vi "Teleop.vi"(10 "Match Info":T1={"Autonomous Elapsed Seconds"=0.0, "TeleOp Elapsed Seconds"=27.581, "Disabled Elapsed Seconds"=153.74, "Visited Autonomous"=FALSE, "Visited TeleOp"=TRUE, "Visited Disabled"=TRUE, "Autonomous Settings"={"Autonomous Style"=enum."Independent", "VI Refnum"=refnum}}, 11 "Call Context":T2=enum."Stop") -> ()   [LabVIEW 2017]
doc: "This VI is called for each enabled TeleOp packet received from the DS. It is typically used to read from joysticks and other inputs and update I/O or setpoints for timed control loops. It should complete and return within 20 milliseconds or risk missing DS packets."
uses:
  <vilib>/Rock Robotics/WPI/DriverStation/WPI_DriverStationDerivedRobotMode.ctl
  <vilib>/Rock Robotics/WPI/DriverStation/WPI_DriverStationMatch Info.ctl
  <vilib>/Rock Robotics/WPI/Utilities/WPI_GetSetVariantRefNum.vi
  Elevator/Implementation/Elevator Published Globals.vi
  <vilib>/Rock Robotics/Network Tables/NT Write Boolean.vi
  Framework/Robot Global Data.vi
  Configuration/Constants.vi
  <vilib>/Rock Robotics/Network Tables/NT Write Numeric Array.vi
  <vilib>/Rock Robotics/Network Tables/NT Write Boolean Array.vi
panel:
  in  "ElevatorheightToSLowMode":dbl=25.0 format="%#_13g"
  in  "OutakeSpeed Fast":dbl=-1.0 format="%#_13g"
  in  "ElevatorInterpolate":cluster{"X":dbl, "Y":dbl}[](array[cluster])=[{"X"=0.0, "Y"=0.0}, {"X"=0.05, "Y"=0.0}, {"X"=0.8, "Y"=0.3}, {"X"=1.0, "Y"=1.0}]
  in  "DisableElevatorSpeed":dbl
  in  "OutakeSens":dbl=0.7
  in  "ElevatorheightToSLowerMode":dbl=45.0 format="%#_13g"
  in  "OutakeSpeed":dbl=-0.7 format="%#_13g"
  in  "IntakeDeadbandFOrOutakeingForTime":dbl=0.06
  in  "Intake Sens":dbl=1.2
  in  "Max dx/dt":dbl=100.0
  in  "Points":cluster{"X":dbl, "Y":dbl}[](array[cluster])=[{"X"=0.0, "Y"=0.0}, {"X"=0.02, "Y"=0.0}, {"X"=0.021, "Y"=0.15}, {"X"=1.0, "Y"=1.0}]
  in  "Drive":enum16{"Cheesy", "Tank"}(ring)
  # "Keep negative"
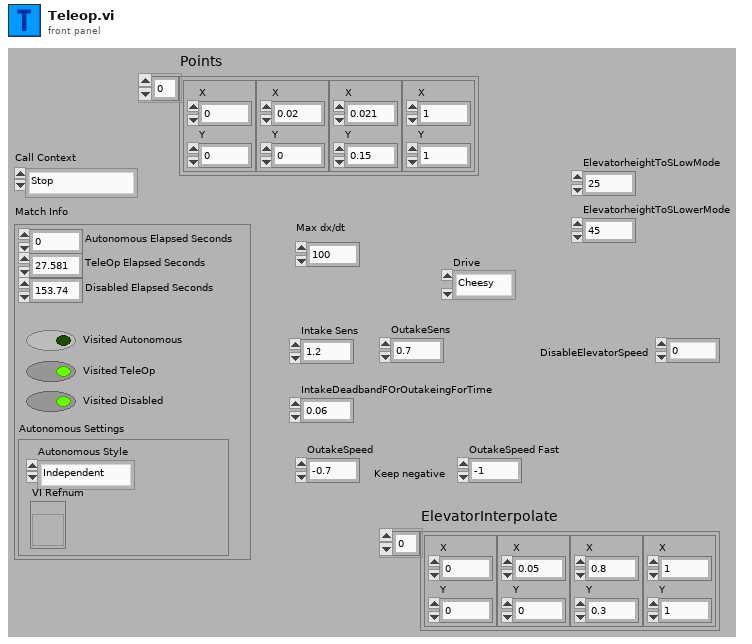
[diagram p1: front panel]
types:
  T1 = typedef "WPI_DriverStationMatch Info.ctl" = cluster{"Autonomous Elapsed Seconds":dbl, "TeleOp Elapsed Seconds":dbl, "Disabled Elapsed Seconds":dbl, "Visited Autonomous":bool, "Visited TeleOp":bool, "Visited Disabled":bool, "Autonomous Settings":cluster{"Autonomous Style":enum16{"Iterative", "Independent"}, "VI Refnum":refnum<vi>}}
  T2 = typedef "WPI_DriverStationDerivedRobotMode.ctl" = enum16{"Init", "Execute", "Stop"}
  T3 = typedef "WPI_JoystickDevRef.ctl" = cluster{"Device":T4}
  T4 = typedef "WPI_JoystickDeviceEnum.ctl" = enum16{"USB 0", "USB 1", "USB 2", "USB 3", "USB 4", "USB 5"}
  T5 = typedef "Command Status Info.ctl" = cluster{"Name":string, "Status":T6, "notifier out":T7}
  T6 = typedef "Completion Status.ctl" = enum16{"Successful", "Aborted", "Incomplete"}
  T7 = typedef "Completion Notifier.ctl" = refnum<notifier>
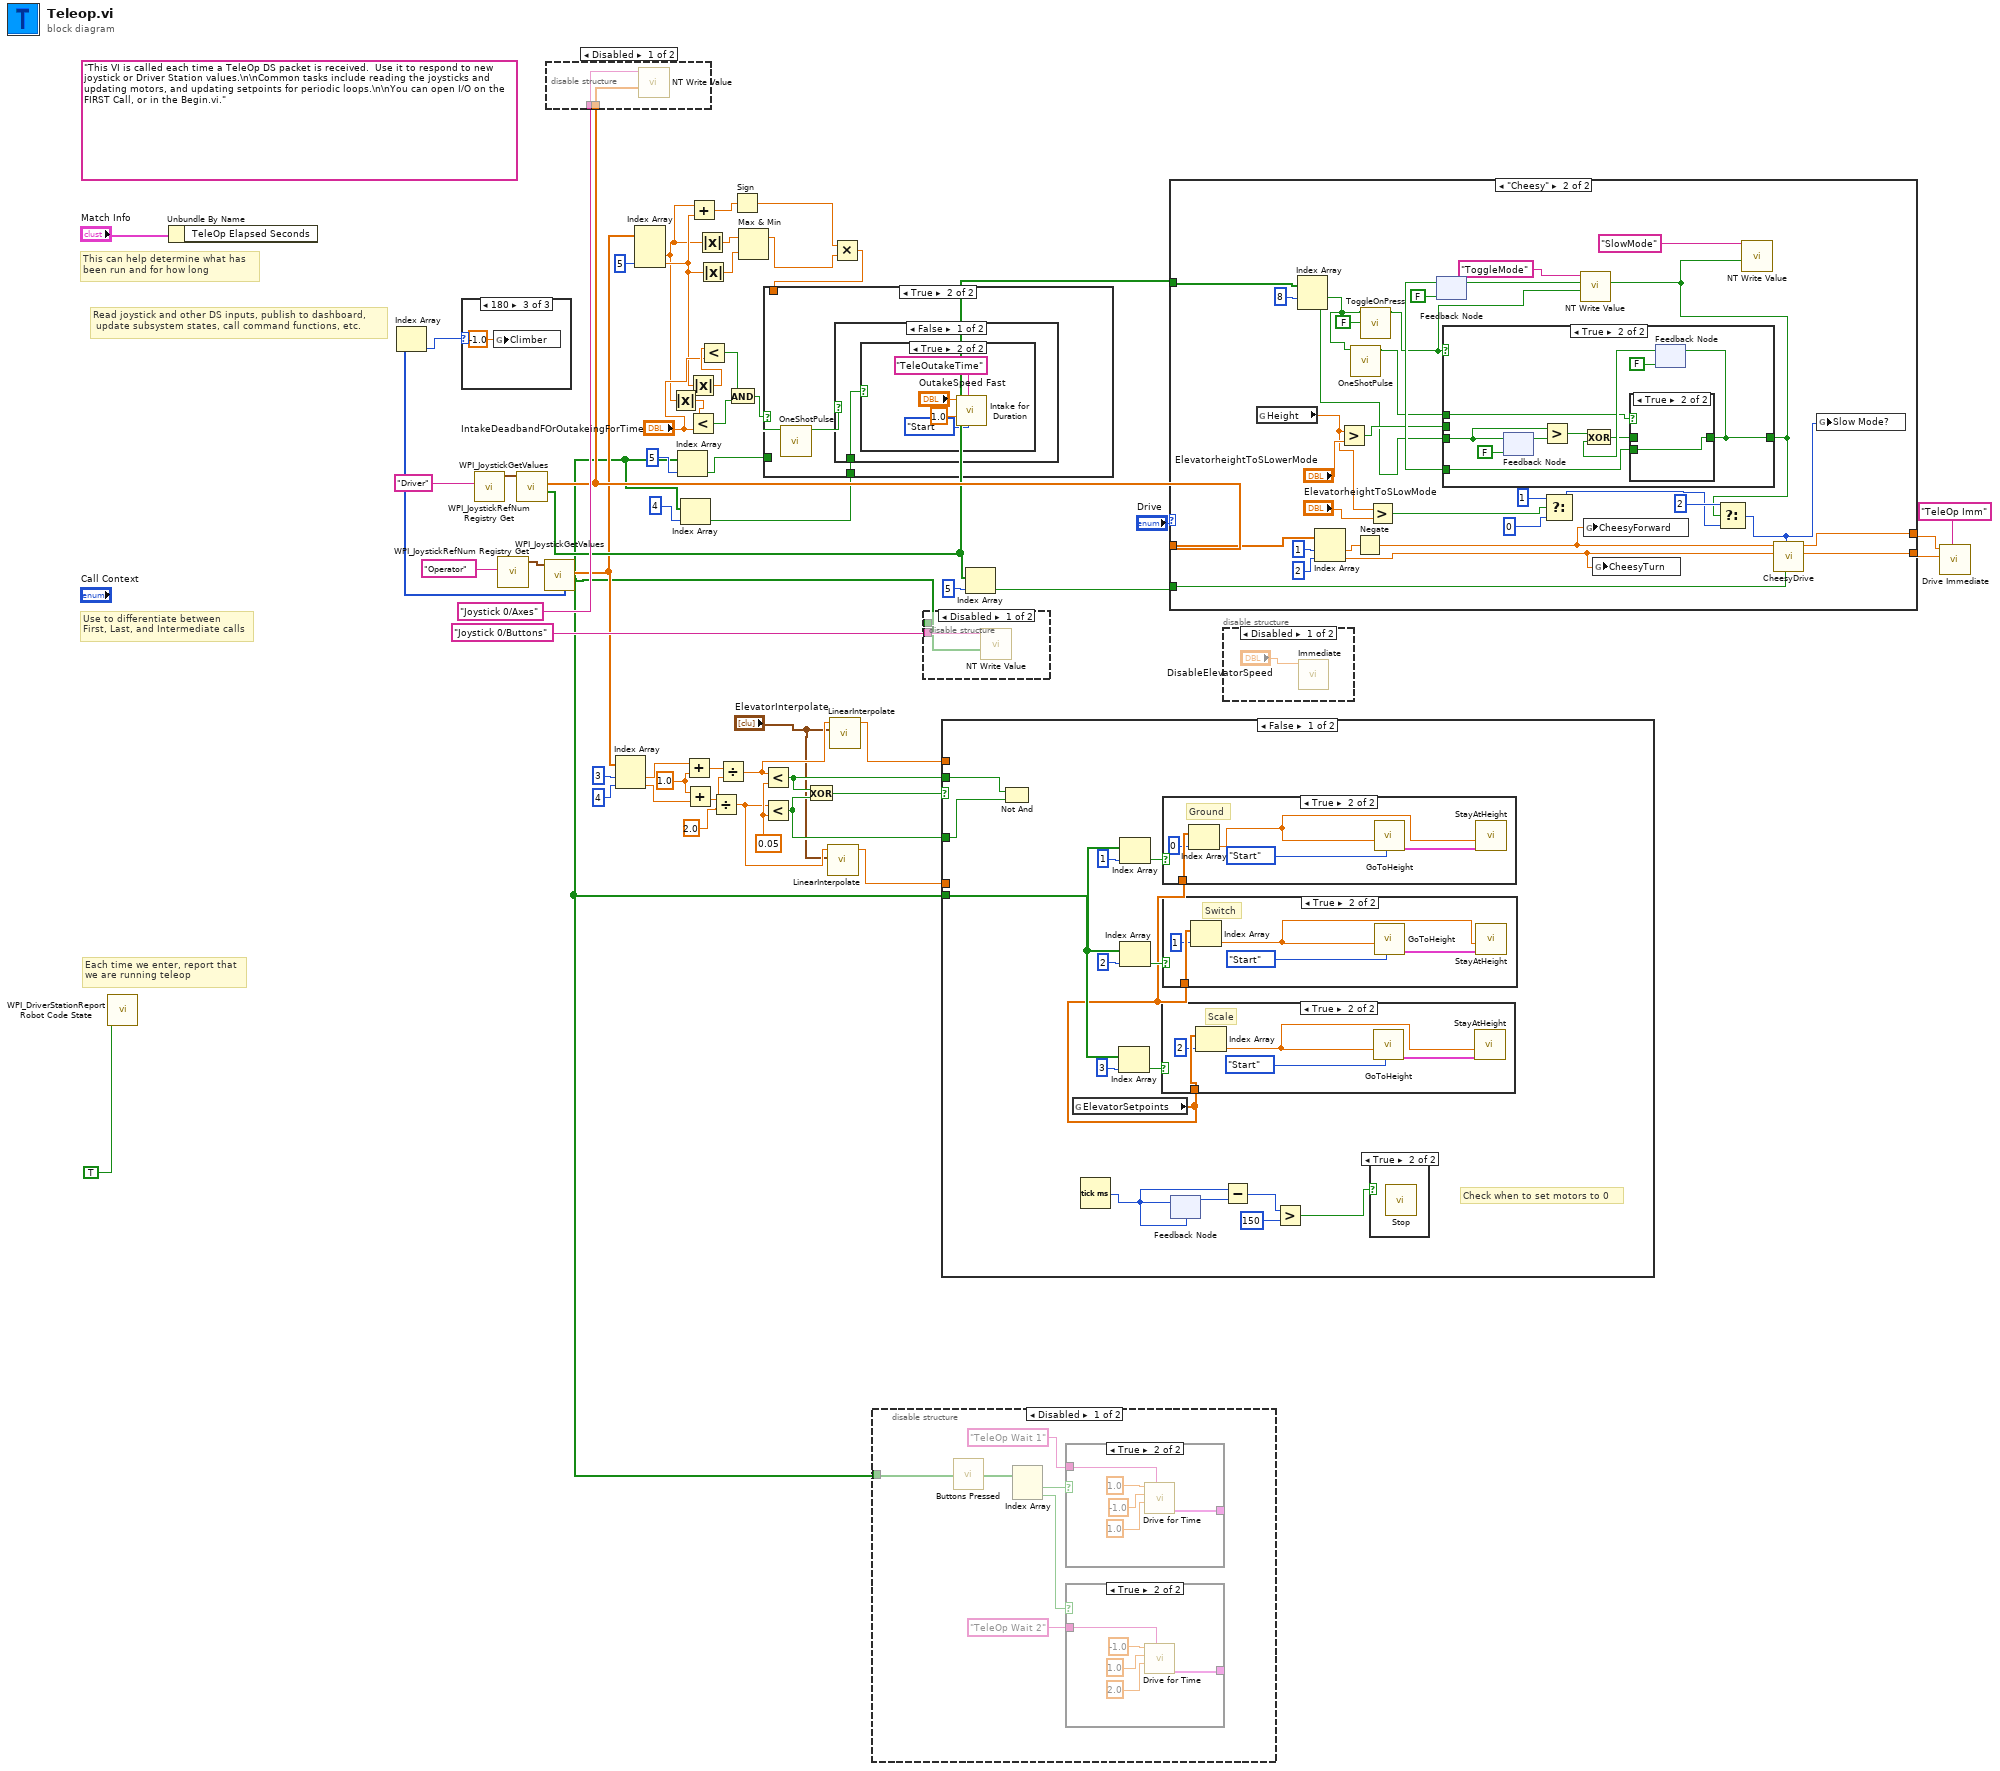
[diagram p0: block diagram]
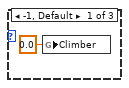
[diagram p2: hidden frame]
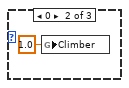
[diagram p3: hidden frame]
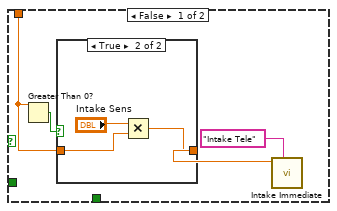
[diagram p5: hidden frame]
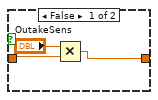
[diagram p6: hidden frame]
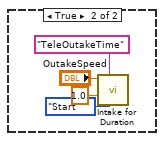
[diagram p8: hidden frame]
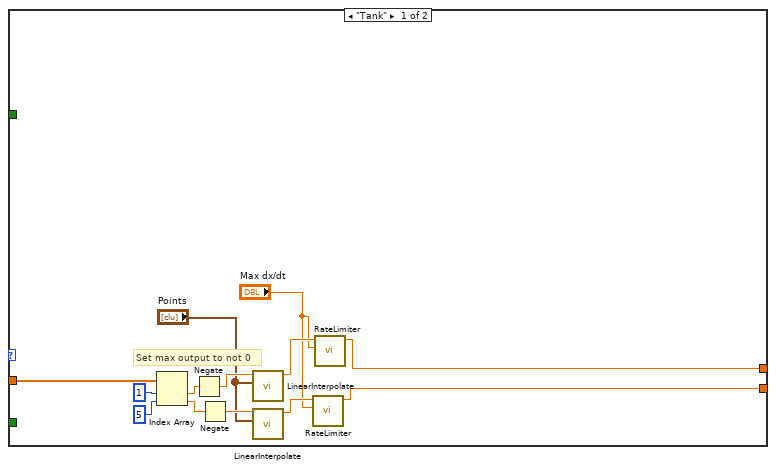
[diagram p11: hidden frame]
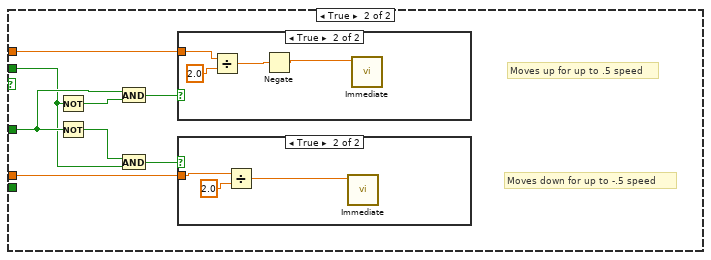
[diagram p18: hidden frame]
diagram:
  w24 = 2.0 ("y")
  w29 = 1.0 ("y")
  w42 = 0.05 ("x")
  (unwired) "This VI is called each time a TeleOp DS packet is received.  Use it to respond to new joystick or Driver Station values.\n\nCommon tasks include reading the joysticks and updating motors, and updating setpoints for periodic loops.\n\nYou can open I/O on the FIRST Call, or in the Begin.vi."
  # "Read joystick and other DS inputs, publish to dashboard,\n update subsystem states, call command functions, etc."
  # "Each time we enter, report that\nwe are running teleop"
  # "Use to differentiate between\nFirst, Last, and Intermediate calls"
  # "This can help determine what has\nbeen run and for how long"
  n1 = call <vilib>:"WPI_DriverStationReport Robot Code State.vi"("TeleOp"=TRUE ("Autonomous")) -> ()  [unwired: 10 in, 1 out]
  n2 = Unbundle By Name("Match Info") -> ()  [unwired: 1 out]
  n3 = call <vilib>:"WPI_JoystickRefNum Registry Get.vi"("refnum name"="Driver") -> ("JoystickDevRef"=w38:T3)  [unwired: 1 in, 9 out]
  n4 = call <vilib>:"WPI_JoystickRefNum Registry Get.vi"("refnum name"="Operator") -> ("JoystickDevRef"=w54:T3)  [unwired: 1 in, 9 out]
  n5 = call <vilib>:"WPI_JoystickGetValues.vi"("JoystickDevRef"=w38) -> ("Buttons"=w35:bool[], "Axes"=w36:dbl[])  [unwired: 6 in, 3 out]
  n6 = call <vilib>:"WPI_JoystickGetValues.vi"("JoystickDevRef"=w54) -> ("Buttons"=w17:bool[], "Axes"=w33:dbl[], "POVs"=w30:i16[])  [unwired: 6 in, 2 out]
  n7 = Index Array(array=w30) -> (element=w1:i16)  [unwired: 1 in]
  n8 = case shown="180" w1 {
    frame -1, Default {
      n9 = global write "Robot Global Data.vi" "Climber"(0.0 ("Climber")) -> ()
    }
    frame 0 {
      n10 = global write "Robot Global Data.vi" "Climber"(1.0 ("Climber")) -> ()
    }
    frame 180 {
      n11 = global write "Robot Global Data.vi" "Climber"(-1.0 ("Climber")) -> ()
    }
  }
  n12 = disable-structure shown="Disabled" {
    disable-tunnel: "Joystick 0/Axes" ("Name") -> [w61 _]
    disable-tunnel: w36 -> [w60 _]
    frame Disabled {
      n13 = call-poly <vilib>:"NT Write Value.vi"("Numeric Array"=w60, "Name"=w61) -> ()  [unwired: 9 in, 1 out]
    }
    frame Enabled {
    }
  }
  n14 = Index Array(array=w33, index #1=3 ("index"), index #2=4 ("index")) -> (element #1=w27:dbl, element #2=w28:dbl)
  n15 = Index Array(array=w33, index #3=5 ("index")) -> (element #2=w6:dbl, element #3=w7:dbl)  [unwired: 2 in, 1 out]
  n16 = Absolute Value(x=w6) -> (abs(x)=w34:dbl)
  n17 = Index Array(array=w17, index=5) -> (element=w31:bool)
  n18 = Index Array(array=w17, index=4) -> (element=w16:bool)
  n19 = Add(x=w27, y=w29) -> (x+y=w26:dbl)
  n20 = Add(x=w29, y=w28) -> (x+y=w25:dbl)
  n21 = Absolute Value(x=w7) -> (abs(x)=w14:dbl)
  n22 = Less?(x=w34, y="IntakeDeadbandFOrOutakeingForTime") -> (x < y?=w12:bool)
  n23 = Add(x=w6, y=w7) -> (x+y=w5:dbl)
  n24 = Absolute Value(x=w6) -> (abs(x)=w9:dbl)
  n25 = Absolute Value(x=w7) -> (abs(x)=w8:dbl)
  n26 = Less?(x=w14, y="IntakeDeadbandFOrOutakeingForTime") -> (x < y?=w11:bool)
  n27 = Divide(x=w25, y=w24) -> (x/y=w21:dbl)
  n28 = Divide(x=w26, y=w24) -> (x/y=w23:dbl)
  n29 = And(x=w11, y=w12) -> (x .and. y?=w10:bool)
  n30 = Sign(1:w5) -> (0:w4:dbl)
  n31 = Max & Min(x=w9, y=w8) -> (max(x,y)=w3:dbl)  [unwired: 1 out]
  n32 = Less?(x=w23, y=w42) -> (x < y?=w41:bool)
  n33 = Less?(x=w21, y=w42) -> (x < y?=w40:bool)
  n34 = Exclusive Or(1:w40, 2:w41) -> (0:w51:bool)
  n35 = call "LinearInterpolate.vi"("Points"="ElevatorInterpolate", "Value"=w21) -> ("Output"=w20:dbl)  [unwired: 9 in]
  n36 = call "LinearInterpolate.vi"("Points"="ElevatorInterpolate", "Value"=w23) -> ("Output"=w22:dbl)  [unwired: 9 in]
  n37 = Multiply(x=w4, y=w3) -> (x*y=w2:dbl)
  n38 = case shown="True" w10 {
    tunnel: w2 -> [w63 _]
    tunnel: w31 -> [_ w74]
    tunnel: w16 -> [_ w72]
    frame False {
      n39 = Greater Than 0?(x=w63) -> (x > 0?=w64:bool)
      n40 = case shown="True" w64 {
        tunnel: w63 -> [w68 w71]
        tunnel: [w66 w70] -> w62
        frame False {
          n41 = Multiply(x="OutakeSens", y=w68) -> (x*y=w66:dbl)
        }
        frame True {
          n42 = Multiply(x="Intake Sens", y=w71) -> (x*y=w70:dbl)
        }
      }
      n43 = call "Intake Immediate.vi"("Description"="Intake Tele", "Speed"=w62) -> ()  [unwired: 9 in, 1 out]
    }
    frame True {
      n44 = call "OneShotPulse.vi"("Input"=w74) -> ("Output"=w73:bool)  [unwired: 10 in]
      n45 = case shown="False" w73 {
        tunnel: w72 -> [w75 _]
        frame False {
          n46 = case shown="True" w75 {
            frame False {
            }
            frame True {
              n47 = call "Intake for Duration.vi"("Synchronization"=enum16{"Start", "Wait"}."Start", "Description"="TeleOutakeTime", "Duration (s)"=1.0, "Speed"="OutakeSpeed Fast") -> ()  [unwired: 7 in, 1 out]
            }
          }
        }
        frame True {
          n48 = call "Intake for Duration.vi"("Synchronization"=enum16{"Start", "Wait"}."Start", "Description"="TeleOutakeTime", "Duration (s)"=1.0, "Speed"="OutakeSpeed") -> ()  [unwired: 7 in, 1 out]
        }
      }
    }
  }
  n49 = disable-structure shown="Disabled" {
    disable-tunnel: w17 -> [w84 _]
    frame Disabled {
      n50 = call "Buttons Pressed.vi"("Button Values"=w84) -> ("Button Presses"=w85:bool[])
      n51 = Index Array(array=w85) -> (element #1=w87:bool, element #2=w86:bool)  [unwired: 2 in]
      n52 = case shown="True" w87 {
        tunnel: [_ w98] -> _
        tunnel: "TeleOp Wait 1" ("Description") -> [_ w97]
        frame False {
        }
        frame True {
          n53 = call "Drive for Time.vi"("Description"=w97, "Seconds"=1.0, "Right Speed"=-1.0, "Left Speed"=1.0) -> ("Command Info Out"=w98:T5)  [unwired: 6 in, 1 out]
        }
      }
      n54 = case shown="True" w86 {
        tunnel: [_ w92] -> _
        tunnel: "TeleOp Wait 2" ("Description") -> [_ w91]
        frame False {
        }
        frame True {
          n55 = call "Drive for Time.vi"("Description"=w91, "Seconds"=2.0, "Right Speed"=1.0, "Left Speed"=-1.0) -> ("Command Info Out"=w92:T5)  [unwired: 6 in, 1 out]
        }
      }
    }
    frame Enabled {
    }
  }
  n56 = disable-structure shown="Disabled" {
    disable-tunnel: "Joystick 0/Buttons" ("Name") -> [w101 _]
    disable-tunnel: w17 -> [w100 _]
    frame Disabled {
      n57 = call-poly <vilib>:"NT Write Value.vi"("Boolean Array"=w100, "Name"=w101) -> ()  [unwired: 9 in, 1 out]
    }
    frame Enabled {
    }
  }
  n58 = case shown="False" w51 {
    tunnel: w17 -> [w116 _]
    tunnel: w41 -> [w110 w134]
    tunnel: w40 -> [w109 w135]
    tunnel: w22 -> [_ w133]
    tunnel: w20 -> [_ w132]
    frame False {
      # "Check when to set motors to 0"
      n59 = Not And(1:w109, 2:w110) -> ()  [unwired: 1 out]
      n60 = global read "Constants.vi" "ElevatorSetpoints"() -> (w102:dbl[])
      n61 = Tick Count (ms)() -> (millisecond timer value=w114:u32)
      n62 = Index Array(array=w116, index=3) -> (element=w103:bool)
      n63 = Index Array(array=w116, index=1) -> (element=w105:bool)
      n64 = Index Array(array=w116, index=2) -> (element=w104:bool)
      n65 = case shown="True" w103 {
        tunnel: w102 -> [_ w119]
        frame False {
        }
        frame True {
          # "Scale"
          n66 = Index Array(array=w119, index=2) -> (element=w118:dbl)
          n67 = call "GoToHeight.vi"("Synchronization"=enum16{"Start", "Wait"}."Start", "Setpoint"=w118) -> ("Command Info Out"=w120:T5)  [unwired: 9 in]
          n68 = call "StayAtHeight.vi"("Command Info In"=w120, "Setpoint"=w118) -> ()  [unwired: 9 in, 1 out]
        }
      }
      n69 = case shown="True" w105 {
        tunnel: w102 -> [_ w129]
        frame False {
        }
        frame True {
          # "Ground"
          n70 = Index Array(array=w129, index=0) -> (element=w128:dbl)
          n71 = call "GoToHeight.vi"("Synchronization"=enum16{"Start", "Wait"}."Start", "Setpoint"=w128) -> ("Command Info Out"=w130:T5)  [unwired: 9 in]
          n72 = call "StayAtHeight.vi"("Command Info In"=w130, "Setpoint"=w128) -> ()  [unwired: 9 in, 1 out]
        }
      }
      n73 = case shown="True" w104 {
        tunnel: w102 -> [_ w124]
        frame False {
        }
        frame True {
          # "Switch"
          n74 = Index Array(array=w124, index=1) -> (element=w123:dbl)
          n75 = call "GoToHeight.vi"("Synchronization"=enum16{"Start", "Wait"}."Start", "Setpoint"=w123) -> ("Command Info Out"=w125:T5)  [unwired: 9 in]
          n76 = call "StayAtHeight.vi"("Command Info In"=w125, "Setpoint"=w123) -> ()  [unwired: 9 in, 1 out]
        }
      }
      n77 = feedback-in #1(w114) -> ()
      n78 = feedback #1(w114) -> (w115:u32)
      n79 = Subtract(x=w114, y=w115) -> (x-y=w113:u32)
      n80 = Greater?(x=w113, y=u32 150) -> (0:w111:bool)
      n81 = case shown="True" w111 {
        frame False {
        }
        frame True {
          n82 = call "Stop.vi"() -> ()  [unwired: 11 in, 1 out]
        }
      }
    }
    frame True {
      # "Moves down for up to -.5 speed"
      # "Moves up for up to .5 speed"
      n83 = Not(x=w134) -> (.not. x?=w136:bool)
      n84 = Not(x=w135) -> (.not. x?=w138:bool)
      n85 = And(x=w135, y=w136) -> (x .and. y?=w137:bool)
      n86 = And(x=w138, y=w134) -> (x .and. y?=w139:bool)
      n87 = case shown="True" w137 {
        tunnel: w133 -> [_ w142]
        frame False {
        }
        frame True {
          n88 = Divide(x=w142, y=2.0) -> (x/y=w141:dbl)
          n89 = Negate(x=w141) -> (-x=w140:dbl)
          n90 = call "Immediate.vi"("Setpoint"=w140) -> ()  [unwired: 10 in, 1 out]
        }
      }
      n91 = case shown="True" w139 {
        tunnel: w132 -> [_ w145]
        frame False {
        }
        frame True {
          n92 = Divide(x=w145, y=2.0) -> (x/y=w144:dbl)
          n93 = call "Immediate.vi"("Setpoint"=w144) -> ()  [unwired: 10 in, 1 out]
        }
      }
    }
  }
  n94 = Index Array(array=w35, index=5) -> (element=w50:bool)
  n95 = case shown="\"Cheesy\"" "Drive" {
    tunnel: w50 -> [_ w187]
    tunnel: [w150 w188] -> w47
    tunnel: [w148 w189] -> w46
    tunnel: w36 -> [w159 w190]
    tunnel: w35 -> [_ w179]
    frame "Tank" {
      # "Set max output to not 0"
      n96 = Index Array(array=w159, index #1=1 ("index"), index #2=5 ("index")) -> (element #1=w156:dbl, element #2=w155:dbl)
      n97 = Negate(x=w156) -> (-x=w154:dbl)
      n98 = Negate(x=w155) -> (-x=w153:dbl)
      n99 = call "LinearInterpolate.vi"("Points"="Points", "Value"=w154) -> ("Output"=w151:dbl)  [unwired: 9 in]
      n100 = call "LinearInterpolate.vi"("Points"="Points", "Value"=w153) -> ("Output"=w149:dbl)  [unwired: 9 in]
      n101 = call "RateLimiter.vi"("Max dx/dt"="Max dx/dt", "Input"=w149) -> ("Output"=w148:dbl)  [unwired: 9 in]
      n102 = call "RateLimiter.vi"("Max dx/dt"="Max dx/dt", "Input"=w151) -> ("Output"=w150:dbl)  [unwired: 9 in]
    }
    frame "Cheesy" {
      n103 = global read "Elevator Published Globals.vi" "Height"() -> (w168:dbl)
      n104 = Index Array(array=w179, index #1=8 ("index")) -> (element #1=w176:bool, element #2=w174:bool)  [unwired: 1 in]
      n105 = Index Array(array=w190, index #1=1 ("index"), index #2=2 ("index")) -> (element #1=w184:dbl, element #2=w169:dbl)
      n106 = Greater?(x=w168, y="ElevatorheightToSLowerMode") -> (0:w175:bool)
      n107 = call "OneShotPulse.vi"("Input"=w176) -> ("Output"=w178:bool)  [unwired: 10 in]
      n108 = Negate(x=w184) -> (-x=w170:dbl)
      n109 = call "ToggleOnPress.vi"("InitialOuput"=FALSE, "Input"=w176) -> ("Output"=w171:bool)  [unwired: 9 in]
      n110 = Greater?(x=w168, y="ElevatorheightToSLowMode") -> (0:w165:bool)
      n111 = feedback #2(FALSE ("InitialOuput")) -> (w181:bool)
      n112 = case shown="True" w171 {
        tunnel: w175 -> [w191 _]
        tunnel: [w191 w194] -> w161
        tunnel: w174 -> [_ w197]
        tunnel: w181 -> [_ w195]
        tunnel: w178 -> [_ w193]
        frame False {
        }
        frame True {
          n113 = feedback #3(FALSE ("Input")) -> (w201:bool)
          n114 = feedback-in #3(w197) -> ()
          n115 = Greater?(x=w197, y=w201) -> (0:w198:bool)
          n116 = feedback #4(FALSE ("InitialOuput")) -> (w199:bool)
          n117 = Exclusive Or(1:w199, 2:w198) -> (0:w196:bool)
          n118 = case shown="True" w193 {
            tunnel: w196 -> [w202 _]
            tunnel: [w202 w203] -> w194
            tunnel: w195 -> [_ w203]
            frame False {
            }
            frame True {
            }
          }
          n119 = feedback-in #4(w194) -> ()
        }
      }
      n120 = feedback-in #2(w161) -> ()
      n121 = Select(t=1, s=w165, f=0 ("index")) -> (s? t:f=w162:i32)
      n122 = call-poly <vilib>:"NT Write Value.vi"("Boolean"=w171, "Name"="ToggleMode") -> ()  [unwired: 9 in, 1 out]
      n123 = global write "Robot Global Data.vi" "CheesyForward"(w170) -> ()
      n124 = global write "Robot Global Data.vi" "CheesyTurn"(w169) -> ()
      n125 = Select(t=2 ("index"), s=w161, f=w162) -> (s? t:f=w160:i32)
      n126 = call-poly <vilib>:"NT Write Value.vi"("Boolean"=w161, "Name"="SlowMode") -> ()  [unwired: 9 in, 1 out]
      n127 = call "CheesyDrive.vi"("Quickturn"=w187, "SlowMode"=w160, "Wheel"=w169, "Throttle"=w170) -> ("Right PWM"=w189:dbl, "Left PWM"=w188:dbl)  [unwired: 6 in]
      n128 = global write "Robot Global Data.vi" "Slow Mode?"(w160) -> ()
    }
  }
  n129 = disable-structure shown="Disabled" {
    frame Disabled {
      n130 = call "Immediate.vi"("Setpoint"="DisableElevatorSpeed") -> ()  [unwired: 10 in, 1 out]
    }
    frame Enabled {
    }
  }
  n131 = call "Drive Immediate.vi"("Description"="TeleOp Imm", "Right Setpoint"=w46, "Left Setpoint"=w47) -> ()  [unwired: 8 in, 1 out]
